vi "Custom Deadbander.vi"(6 "Invert (TF)":bool, 8 "y":dbl, 11 "x":dbl) -> (0 "y edited":dbl, 3 "X edited":dbl)   [LabVIEW 2012]
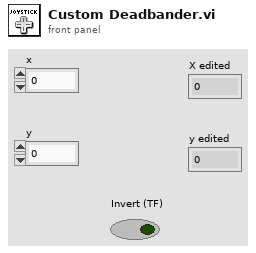
[diagram p1: front panel]
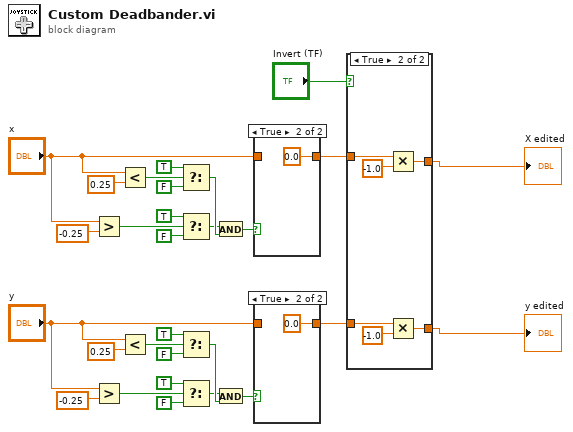
[diagram p0: block diagram]
diagram:
  n1 = Greater?(x="x", y=-0.25) -> (0:w29:bool)
  n2 = Greater?(x="y", y=-0.25) -> (0:w17:bool)
  n3 = Less?(x="x", y=0.25) -> (x < y?=w26:bool)
  n4 = Less?(x="y", y=0.25) -> (x < y?=w14:bool)
  n5 = Select(t=TRUE, s=w26, f=FALSE) -> (s? t:f=w23:bool)
  n6 = Select(t=TRUE, s=w29, f=FALSE) -> (s? t:f=w22:bool)
  n7 = Select(t=TRUE, s=w14, f=FALSE) -> (s? t:f=w11:bool)
  n8 = Select(t=TRUE, s=w17, f=FALSE) -> (s? t:f=w10:bool)
  n9 = And(x=w22, y=w23) -> (x .and. y?=w19:bool)
  n10 = And(x=w10, y=w11) -> (x .and. y?=w7:bool)
  n11 = case shown="True" w19 {
    tunnel: "x" -> [w30 _]
    tunnel: [w30 0.0] -> w4
    frame False {
    }
    frame True {
    }
  }
  n12 = case shown="True" w7 {
    tunnel: "y" -> [w32 _]
    tunnel: [w32 0.0] -> w3
    frame False {
    }
    frame True {
    }
  }
  n13 = case shown="True" "Invert (TF)" {
    tunnel: w4 -> [w35 w37]
    tunnel: [w35 w36] -> w1
    tunnel: w3 -> [w34 w39]
    tunnel: [w34 w38] -> w2
    frame False {
    }
    frame True {
      n14 = Multiply(x=w37, y=-1.0) -> (x*y=w36:dbl)
      n15 = Multiply(x=w39, y=-1.0) -> (x*y=w38:dbl)
    }
  }
  "X edited" <- w1
  "y edited" <- w2
